vi "VI Tree.vi"   [LabVIEW 2009, in "Keithley 24XX.lvlib"]
doc: "This is the instrument driver for the Keithley 2400 Series SourceMeter. The VI Tree displays all the user-callable VIs of the instrument driver in an organized table."
uses:
  <instrlib>/Keithley 24XX/Keithley 24XX.lvlib
  <instrlib>/Keithley 24XX/Public/Data/Read (Math).vi
  <instrlib>/Keithley 24XX/Public/Data/Read (Statistical).vi
  <instrlib>/Keithley 24XX/Public/Data/Read (Multiple Points).vi
  <instrlib>/Keithley 24XX/Public/Data/Read (Single Point).vi
  <instrlib>/Keithley 24XX/Public/Data/Low Level/Fetch (Measurements).vi
panel:
  # "(c) 2006 National Instruments.  ALL RIGHTS RESERVED."
  # "SEE DIAGRAM\nFOR VI TREE."
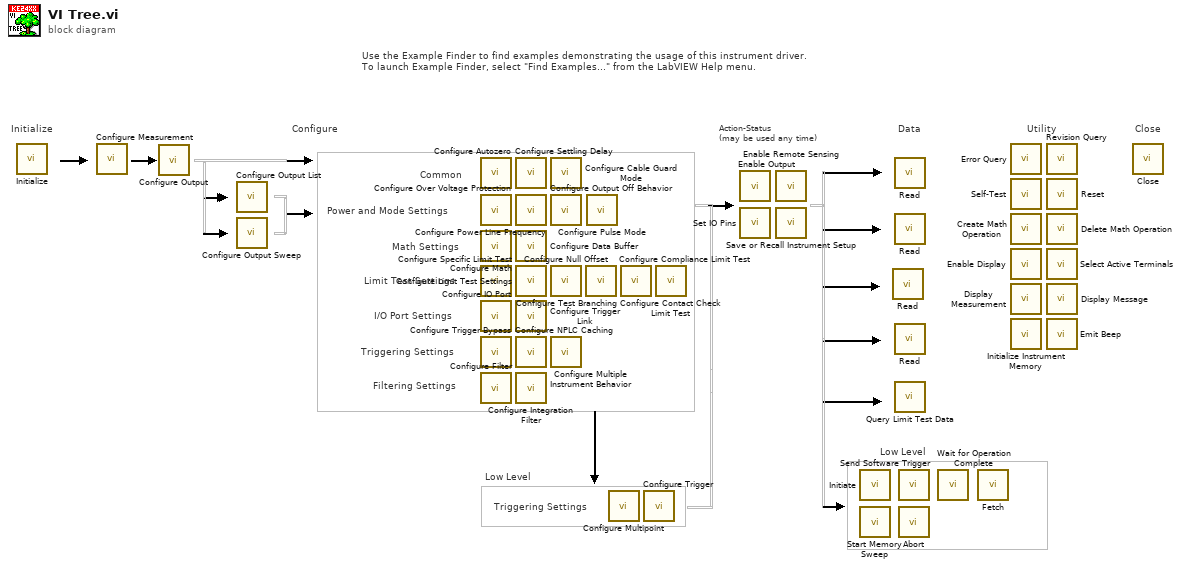
[diagram p0: block diagram]
diagram:
  # "Triggering Settings"
  # "Low Level"
  # "Action-Status\n(may be used any time)"
  # "Filtering Settings"
  # "Triggering Settings"
  # "Power and Mode Settings"
  # "Math Settings"
  # "Limit Test Settings"
  # "I/O Port Settings"
  # "Common"
  # "Low Level"
  # "Use the Example Finder to find examples demonstrating the usage of this instrument driver.\nTo launch Example Finder, select \"Find Examples...\" from the LabVIEW Help menu."
  # "Configure"
  # "Utility"
  # "Data"
  # "Close"
  # "Initialize"
  n1 = call <instrlib>:"Initialize.vi"() -> ()  [unwired: 10 in, 2 out]
  n2 = call <instrlib>:"Configure Measurement.vi"() -> ()  [unwired: 10 in, 2 out]
  n3 = call <instrlib>:"Configure Output.vi"() -> ()  [unwired: 10 in, 2 out]
  n4 = call <instrlib>:"Configure Output List.vi"() -> ()  [unwired: 10 in, 2 out]
  n5 = call <instrlib>:"Configure Output Sweep.vi"() -> ()  [unwired: 14 in, 2 out]
  n6 = call <instrlib>:"Configure Autozero.vi"() -> ()  [unwired: 10 in, 2 out]
  n7 = call <instrlib>:"Configure Over Voltage Protection.vi"() -> ()  [unwired: 10 in, 2 out]
  n8 = call <instrlib>:"Configure Math.vi"() -> ()  [unwired: 10 in, 2 out]
  n9 = call <instrlib>:"Configure Specific Limit Test.vi"() -> ()  [unwired: 14 in, 2 out]
  n10 = call <instrlib>:"Configure IO Port.vi"() -> ()  [unwired: 10 in, 2 out]
  n11 = call <instrlib>:"Configure Trigger Bypass.vi"() -> ()  [unwired: 10 in, 2 out]
  n12 = call <instrlib>:"Configure Filter.vi"() -> ()  [unwired: 10 in, 2 out]
  n13 = call <instrlib>:"Configure Settling Delay.vi"() -> ()  [unwired: 10 in, 2 out]
  n14 = call <instrlib>:"Configure Power Line Frequency.vi"() -> ()  [unwired: 10 in, 2 out]
  n15 = call <instrlib>:"Configure Data Buffer.vi"() -> ()  [unwired: 10 in, 2 out]
  n16 = call <instrlib>:"Configure Limit Test Settings.vi"() -> ()  [unwired: 10 in, 2 out]
  n17 = call <instrlib>:"Configure Trigger Link.vi"() -> ()  [unwired: 14 in, 2 out]
  n18 = call <instrlib>:"Configure NPLC Caching.vi"() -> ()  [unwired: 10 in, 2 out]
  n19 = call <instrlib>:"Configure Integration Filter.vi"() -> ()  [unwired: 10 in, 2 out]
  n20 = call <instrlib>:"Configure Cable Guard Mode.vi"() -> ()  [unwired: 10 in, 2 out]
  n21 = call <instrlib>:"Configure Output Off Behavior.vi"() -> ()  [unwired: 10 in, 2 out]
  n22 = call <instrlib>:"Configure Null Offset.vi"() -> ()  [unwired: 10 in, 2 out]
  n23 = call <instrlib>:"Configure Multiple Instrument Behavior.vi"() -> ()  [unwired: 10 in, 2 out]
  n24 = call <instrlib>:"Configure Test Branching.vi"() -> ()  [unwired: 10 in, 2 out]
  n25 = call <instrlib>:"Configure Pulse Mode.vi"() -> ()  [unwired: 10 in, 2 out]
  n26 = call <instrlib>:"Configure Multipoint.vi"() -> ()  [unwired: 10 in, 2 out]
  n27 = call <instrlib>:"Configure Compliance Limit Test.vi"() -> ()  [unwired: 10 in, 2 out]
  n28 = call <instrlib>:"Configure Trigger.vi"() -> ()  [unwired: 10 in, 2 out]
  n29 = call <instrlib>:"Configure Contact Check Limit Test.vi"() -> ()  [unwired: 10 in, 2 out]
  n30 = call <instrlib>:"Enable Output.vi"() -> ()  [unwired: 10 in, 2 out]
  n31 = call <instrlib>:"Set IO Pins.vi"() -> ()  [unwired: 10 in, 2 out]
  n32 = call <instrlib>:"Enable Remote Sensing.vi"() -> ()  [unwired: 10 in, 2 out]
  n33 = call <instrlib>:"Save or Recall Instrument Setup.vi"() -> ()  [unwired: 10 in, 2 out]
  n34 = call <instrlib>:"Initiate.vi"() -> ()  [unwired: 10 in, 2 out]
  n35 = call <instrlib>:"Start Memory Sweep.vi"() -> ()  [unwired: 10 in, 2 out]
  n36 = call-poly <instrlib>:"Read.vi"() -> ()  [unwired: 13 in, 3 out]
  n37 = call-poly <instrlib>:"Read.vi"() -> ()  [unwired: 9 in, 7 out]
  n38 = call-poly <instrlib>:"Read.vi"() -> ()  [unwired: 9 in, 7 out]
  n39 = call-poly <instrlib>:"Read.vi"() -> ()  [unwired: 13 in, 3 out]
  n40 = call <instrlib>:"Query Limit Test Data.vi"() -> ()  [unwired: 9 in, 3 out]
  n41 = call <instrlib>:"Send Software Trigger.vi"() -> ()  [unwired: 10 in, 2 out]
  n42 = call <instrlib>:"Abort.vi"() -> ()  [unwired: 10 in, 2 out]
  n43 = call <instrlib>:"Wait for Operation Complete.vi"() -> ()  [unwired: 10 in, 2 out]
  n44 = call-poly <instrlib>:"Fetch.vi"() -> ()  [unwired: 9 in, 7 out]
  n45 = call <instrlib>:"Error Query.vi"() -> ()  [unwired: 8 in, 4 out]
  n46 = call <instrlib>:"Self-Test.vi"() -> ()  [unwired: 8 in, 4 out]
  n47 = call <instrlib>:"Create Math Operation.vi"() -> ()  [unwired: 10 in, 2 out]
  n48 = call <instrlib>:"Enable Display.vi"() -> ()  [unwired: 10 in, 2 out]
  n49 = call <instrlib>:"Display Measurement.vi"() -> ()  [unwired: 10 in, 2 out]
  n50 = call <instrlib>:"Initialize Instrument Memory.vi"() -> ()  [unwired: 10 in, 2 out]
  n51 = call <instrlib>:"Revision Query.vi"() -> ()  [unwired: 8 in, 4 out]
  n52 = call <instrlib>:"Reset.vi"() -> ()  [unwired: 10 in, 2 out]
  n53 = call <instrlib>:"Delete Math Operation.vi"() -> ()  [unwired: 10 in, 2 out]
  n54 = call <instrlib>:"Select Active Terminals.vi"() -> ()  [unwired: 10 in, 2 out]
  n55 = call <instrlib>:"Display Message.vi"() -> ()  [unwired: 10 in, 2 out]
  n56 = call <instrlib>:"Emit Beep.vi"() -> ()  [unwired: 10 in, 2 out]
  n57 = call <instrlib>:"Close.vi"() -> ()  [unwired: 11 in, 1 out]
